vi "Clear Connection Control by Reference.vi"(8 "error in":errorcluster, 11 "Channel Connection":refnum<vi>) -> (0 "error out":errorcluster)   [LabVIEW 2021, in "CIF_UI.lvclass"]
uses:
  Typedef/Channel Connection.ctl
  CIF_UI.lvclass
  CIF_UI.lvclass/CIF_UI.ctl
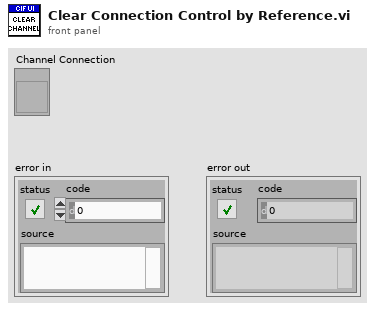
[diagram p1: front panel]
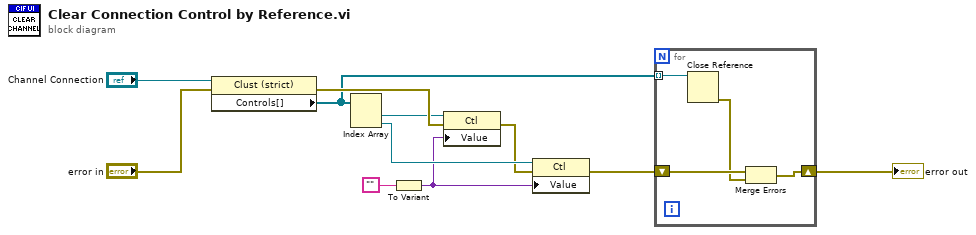
[diagram p0: block diagram]
diagram:
  n1 = property class="Clust (strict)"(reference="Channel Connection", error in="error in") -> (error out=w8:errorcluster, "Controls[]"=w2:refnum<vi>[])  [unwired: 1 out]
  n2 = Index Array(array=w2) -> (element #1=w7:refnum<vi>, element #2=w6:refnum<vi>)  [unwired: 2 in]
  n3 = To Variant(anything="") -> (Variant=w5:variant)
  n4 = property class="Ctl"(reference=w7, error in=w8, "Value"=w5) -> (error out=w3:errorcluster)  [unwired: 1 out]
  n5 = property class="Ctl"(reference=w6, error in=w3, "Value"=w5) -> (error out=w1:errorcluster)  [unwired: 1 out]
  n6 = for {
    tunnel: w2 -> [w15] mode=indexing
    shift-right: [w12] -> w11
    shift-left: w1 -> [w14]
    n7 = Close Reference(reference=w15) -> (error out=w13:errorcluster)  [unwired: 1 in]
    n8 = Merge Errors(w14, w13) -> (w12:errorcluster)
  }
  "error out" <- w11
